vi "getREFconfig.vi"(8 "error in (no error)":errorcluster, 11 "Instrument.Lockin in":refnum<class "Instrument.Lockin.lvclass">) -> (0 "error out":errorcluster, 2 "REFconfig":T1=[{"Enable?"=FALSE, "Channel"=13, "Frequency"=0.1, "Phase"=0.0, "TC"=1e-05, "Roll-Off"=1}] {"Roll-Off" min=1; "TC" min=0.0001 format="%#_3p"; "Phase" format="%#_3g"; "Frequency" min=0.0001 max=200000.0 format="%#_6p"; "Channel" min=1}, 3 "Instrument.Lockin out":refnum<class "Instrument.Lockin.lvclass">)   [LabVIEW 2019, in "Instrument.Lockin.lvlib" / "Instrument.Lockin.lvclass"]
doc: "API to get the results of lockin calculation.\n\nIf address=\"\", this API reads from localhost\nIf address is remote lockin, you need to add this computer to allowed whitelist on the lockin computer you are trying to access."
uses:
  Instrument.Lockin.lvclass
  Instrument.DAQ/Typedefs/REF.Channel--Cluster--Array.ctl
  Instrument.DAQ/Typedefs/REF.Channel--Cluster.ctl
  Typedefs/API/Lockin.Commands--Enum.ctl
  4b9412f8-f7b6-4d45-bf9e-37bf450d4a45.vi
  4b9412f8-f7b6-4d45-bf9e-37bf450d4a45.vi/6566a676-9d5a-48d5-b563-53afd2a5f791.vi
  4b9412f8-f7b6-4d45-bf9e-37bf450d4a45.vi/3b0bf875-f50f-4477-a83f-6b9df75c66bb.vi
  <vilib>/Utility/Data Type/Get Type Information.vi
  <vilib>/JDP Science/JSONtext/JSON text to Variant.vi
  <vilib>/JDP Science/JSONtext/LVClass Serializer/JSONtext LVClass Serializer.lvclass
  Instrument.DAQ/Instrument.DAQ.lvclass
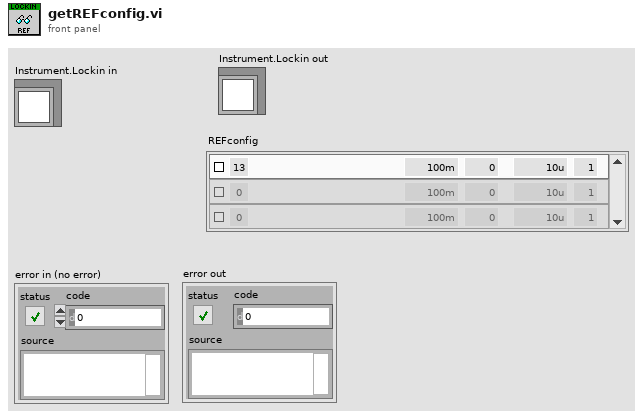
[diagram p1: front panel]
types:
  T1 = typedef "Instrument.Lockin.lvlib/Instrument.DAQ.lvclass/REF.Channel--Cluster--Array.ctl" = T2[]
  T2 = typedef "Instrument.Lockin.lvlib/Instrument.DAQ.lvclass/REF.Channel--Cluster.ctl" = cluster{"Enable?":bool, "Channel":i32, "Frequency":dbl, "Phase":dbl, "TC":dbl, "Roll-Off":i32}
  T3 = typedef "Instrument.Lockin.lvlib/Instrument.Lockin.lvclass/Lockin.Commands--Enum.ctl" = enum16{"setAO", "setAO_Amplitude", "setAO_DC", "setAO_Frequency", "setAO_Phase", "setAO_Function", "setREF", "setREF_Frequency", "setREF_Phase", "setREF_TC", "setREF_Roll-Off", "setDAQ", "setSampling", "setState", "getState", "getAO", "getAI", "getResults", "getSampling", "getAOconfig", "getREFconfig", "setInputGain", "setOutputGain", "getInputGain", "getOutputGain", "setSamplingFsMode", "getSamplingFsMode", "setSweep", "setSweep_Time", "setSweep_Table", "getStatus", "getSweepResults", "getSweepWaveforms", "logConfiguration", "startLogging", "stopLogging"}
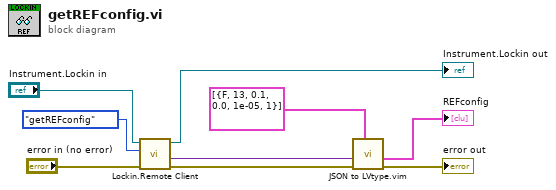
[diagram p0: block diagram]
diagram:
  n1 = call "Lockin.Remote Client.vi"("error in (no error)"="error in (no error)", "Command"=Lockin.Commands--Enum."getREFconfig", "Instrument.Lockin in"="Instrument.Lockin in") -> ("error out"=w6:errorcluster, "Data out"=w3:variant, "Instrument.Lockin out"=→"Instrument.Lockin out":refnum<class "Instrument.Lockin.lvclass">)  [unwired: 6 in]
  n2 = call "JSON to LVtype.vim"("type"=T1 [{"Enable?"=FALSE, "Channel"=13, "Frequency"=0.1, "Phase"=0.0, "TC"=1e-05, "Roll-Off"=1}] ("REFconfig"), "error in (no error)"=w6, "JSON Data in"=w3) -> ("error out"=→"error out":errorcluster, "Data out"=→"REFconfig":T2[])  [unwired: 7 in]
